vi "2d Gaussian array.vi"() -> (3 "Intensity Graph":u16[][](graph))   [LabVIEW 2020]
uses:
  NI_PtbyPt.lvlib
panel:
  in  "wx":u8=255
  in  "wy":u8=150
  in  "No spot sizes x":dbl=7.0 format="%.3f"
  in  "A":dbl=4095.0
  in  "add noise":bool
  out "Numeric 2":i32
  out "Numeric":i32
  in  "only noise":bool
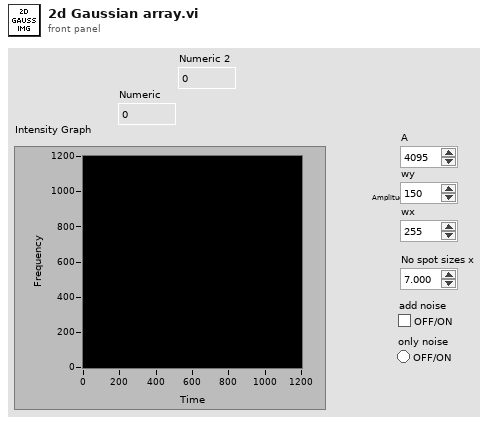
[diagram p1: front panel]
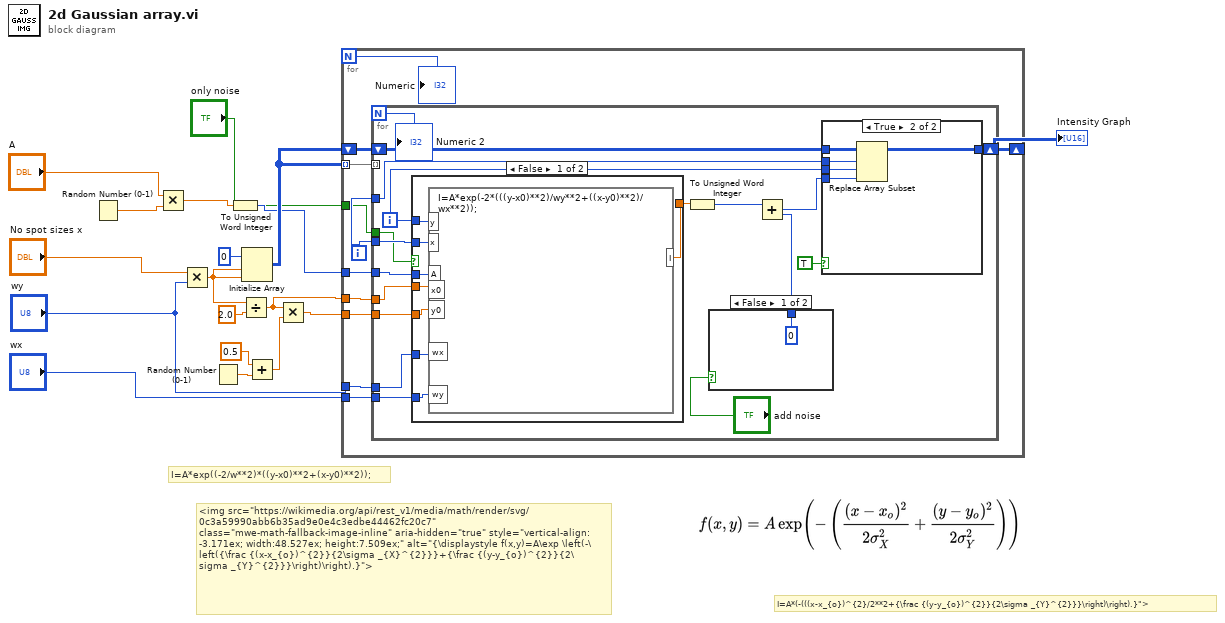
[diagram p0: block diagram]
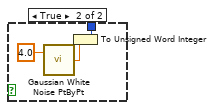
[diagram p2: hidden frame]
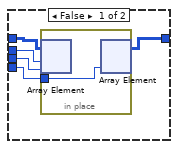
[diagram p3: hidden frame]
diagram:
  # "I=A*(-(((x-x_{o})^{2}/2**2+{\\frac {(y-y_{o})^{2}}{2\\sigma _{Y}^{2}}}\\right)\\right).}\">"
  # "<img src=\"https://wikimedia.org/api/rest_v1/media/math/render/svg/0c3a59990abb6b35ad9e0e4c3edbe44462fc20c7\" class=\"mwe-math-fallback-image-inline\" aria-hidden=\"true\" style=\"vertical-align: -3.171ex; width:48.527ex; height:7.509ex;\" alt=\"{\\displaystyle f(x,y)=A\\exp \\left(-\\left({\\frac {(x-x_{o})^{2}}{2\\sigma _{X}^{2}}}+{\\frac {(y-y_{o})^{2}}{2\\sigma _{Y}^{2}}}\\right)\\right).}\">"
  # "I=A*exp((-2/w**2)*((y-x0)**2+(x-y0)**2));"
  n1 = Random Number (0-1)() -> (number: 0 to 1=w2:dbl)
  n2 = Multiply(x="A", y=w2) -> (x*y=w5:dbl)
  n3 = Multiply(x="No spot sizes x", y="wy") -> (x*y=w8:dbl)
  n4 = Random Number (0-1)() -> (number: 0 to 1=w13:dbl)
  n5 = To Unsigned Word Integer(number=w5) -> (unsigned 16bit integer=w4:u16)
  n6 = Divide(x=w8, y=2.0) -> (x/y=w16:dbl)
  n7 = Initialize Array(u16 0 ("element"), w8, w8) -> (w11:u16[][])
  n8 = Add(x=0.5, y=w13) -> (x+y=w15:dbl)
  n9 = Multiply(x=w16, y=w15) -> (x*y=w17:dbl)
  n10 = for {
    N -> [w20]
    tunnel: w11 -> [w29] mode=indexing
    shift-right: [w27] -> w6
    shift-left: w11 -> [w28]
    tunnel: w4 -> [w26]
    tunnel: w16 -> [w24]
    tunnel: "wy" -> [w23]
    tunnel: w17 -> [w22]
    tunnel: "only noise" -> [w21]
    tunnel: "wx" -> [w19]
    i -> [w25]
    n11 = for {
      N -> [w36]
      tunnel: w29 -> [_] mode=indexing
      shift-right: [w46] -> w27
      shift-left: w28 -> [w47]
      tunnel: w25 -> [w45]
      tunnel: w26 -> [w43]
      tunnel: w25 -> [w42]
      tunnel: w24 -> [w41]
      tunnel: w23 -> [w40]
      tunnel: w22 -> [w39]
      tunnel: w21 -> [w37]
      tunnel: w19 -> [w30]
      i -> [w44]
      n12 = case shown="False" w37 {
        tunnel: w44 -> [w70 _]
        tunnel: w43 -> [w69 _]
        tunnel: w42 -> [w68 _]
        tunnel: w41 -> [w67 _]
        tunnel: w40 -> [w66 _]
        tunnel: w39 -> [w65 _]
        tunnel: [w64 _] -> w33
        tunnel: w30 -> [w63 _]
        frame False {
          n13 = formula code="I=A*exp(-2*(((y-x0)**2)/wy**2+((x-y0)**2)/wx**2));"("y"=w70, "A"=w69, "x0"=w67, "x"=w68, "wx"=w66, "y0"=w65, "wy"=w63) -> ("I"=w64:dbl)
        }
        frame True {
        }
      }
      n14 = To Unsigned Word Integer(number=w33) -> (unsigned 16bit integer=w32:u16)
      n15 = case shown="False" "add noise" {
        tunnel: [u16 0 w49] -> w34
        frame False {
        }
        frame True {
          n16 = call "Gaussian White Noise PtByPt.vi"("standard deviation"=4.0) -> ("Gaussian white noise"=w50:dbl)  [unwired: 2 in]
          n17 = To Unsigned Word Integer(number=w50) -> (unsigned 16bit integer=w49:u16)
        }
      }
      n18 = Add(x=w32, y=w34) -> (x+y=w38:u16)
      n19 = case shown="True" TRUE {
        tunnel: w47 -> [w56 w62]
        tunnel: [w55 w61] -> w46
        tunnel: w45 -> [w54 w60]
        tunnel: w44 -> [w53 w59]
        tunnel: w38 -> [w52 w58]
        frame False {
          n20 = in-place {
            in-place-border: w52 -> [w57]
            n21 = in-place-array #1(w56, w54, w53) -> ()  [unwired: 1 out]
            n22 = in-place-array #1(w57) -> (w55:u16[][])  [unwired: 2 out]
          }
        }
        frame True {
          n23 = Replace Array Subset(array=w62, new element=w58, index (row)=w60, index (col)=w59) -> (w61:u16[][])
        }
      }
      "Numeric 2" <- w36
    }
    "Numeric" <- w20
  }
  "Intensity Graph" <- w6
